vi "final.vi"() -> ()   [LabVIEW 2014]
panel:
  in  "start":bool
  out "Boolean":bool
  out "Score":i32
  out "XY Graph":cluster{dbl[], dbl[]}[](graph)
  in  "Width":dbl=6.0
  in  "stop":bool
  in  "UP":bool
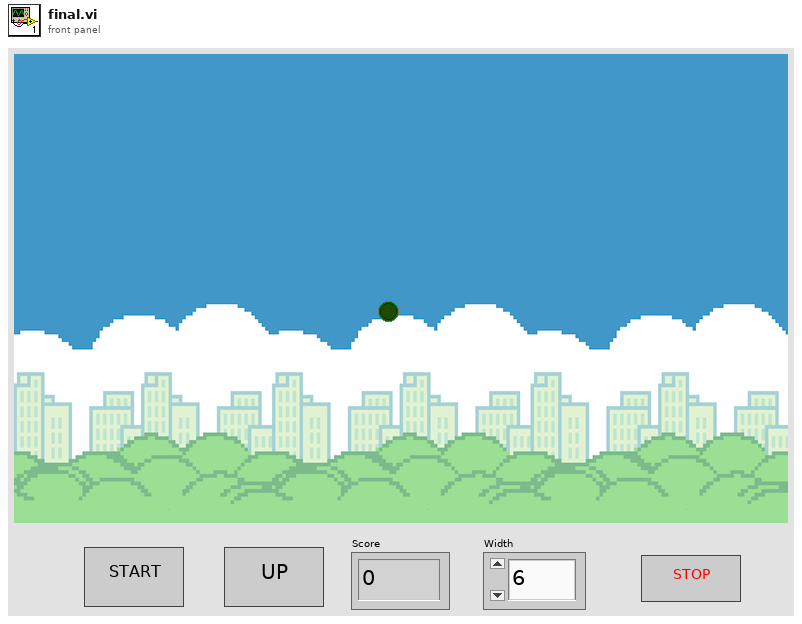
[diagram p1: front panel]
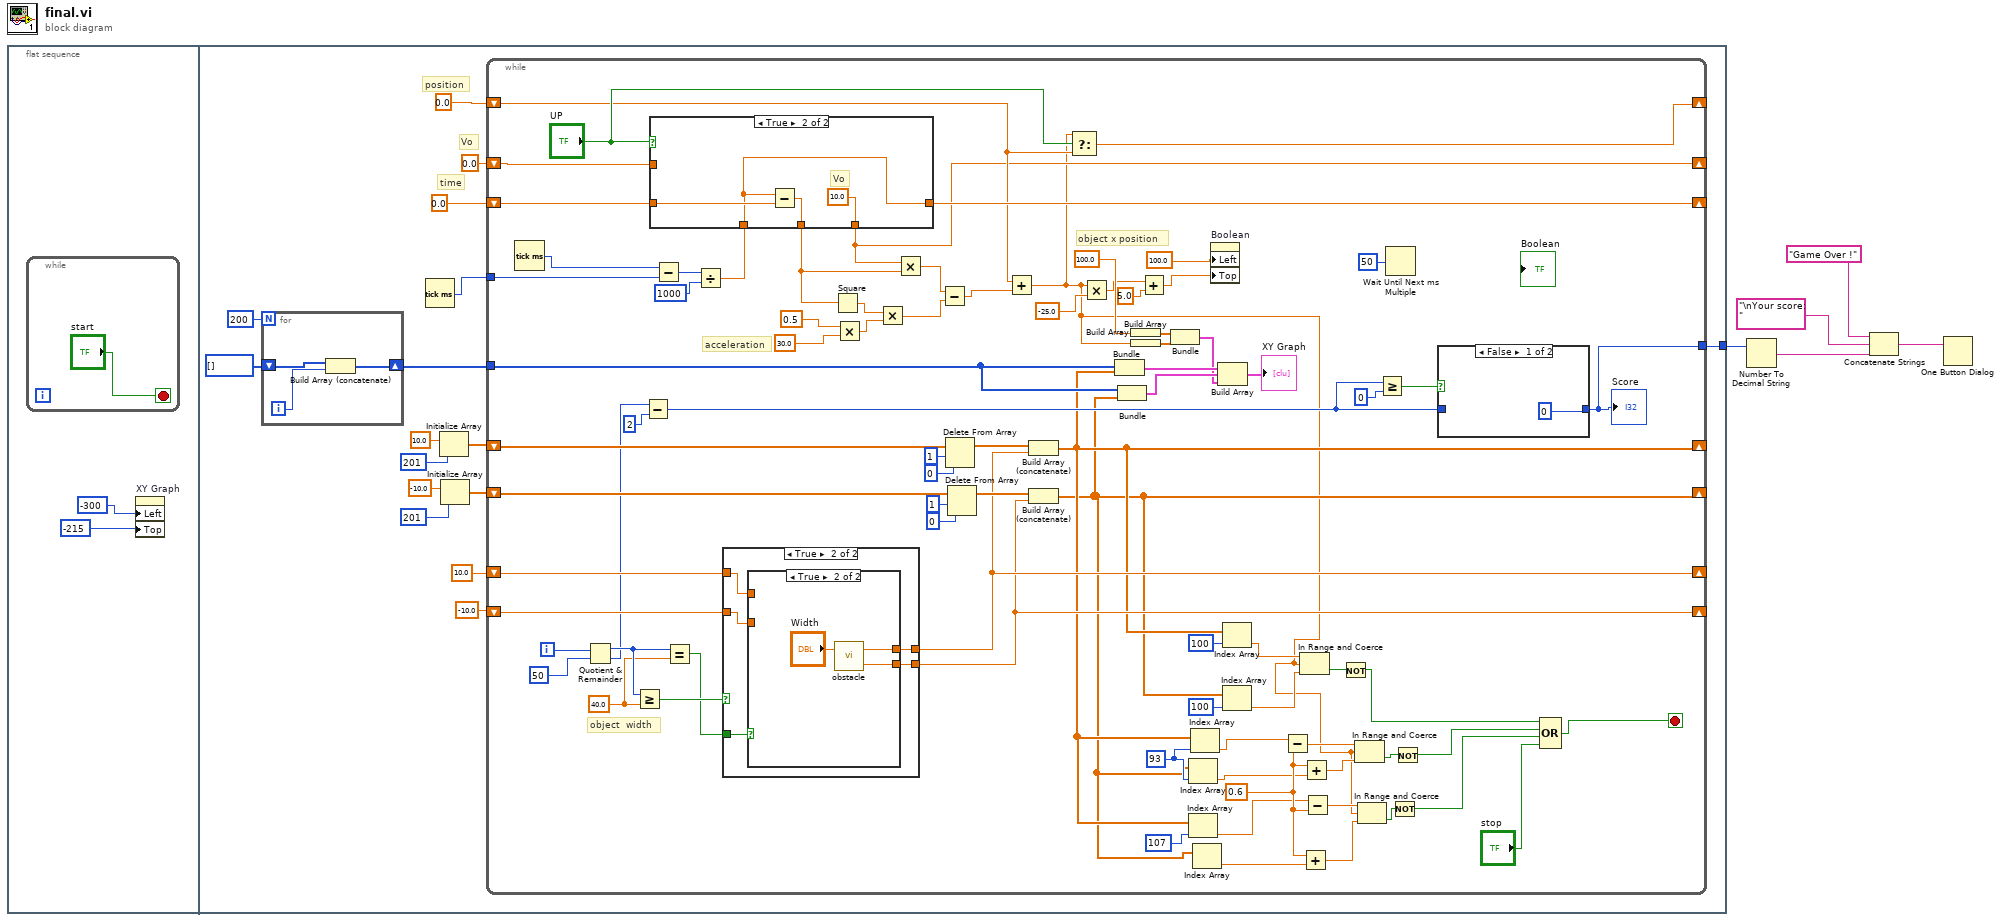
[diagram p0: block diagram]
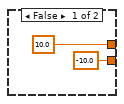
[diagram p3: hidden frame]
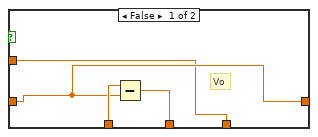
[diagram p5: hidden frame]
diagram:
  n1 = flat-sequence {
    tunnel: [w9] -> w4
    frame #0 {
      n2 = while {
        stop <- "start" stop-if-true
      }
      n3 = property on="XY Graph" class="XYGraph (strict)"("Left"=-300 ("Position:Left"), "Top"=-215 ("Position:Top")) -> ()  [unwired: 2 in, 2 out]
    }
    frame #1 {
      # "Vo"
      # "position"
      # "time"
      n4 = for {
        N: 200 -> [_]
        shift-right: [w25] -> w11
        shift-left: i32[] [] -> [w27]
        i -> [w26]
        n5 = Build Array (concatenate)(w27, w26) -> (w25:i32[])
      }
      n6 = Tick Count (ms)() -> (millisecond timer value=w22:u32)
      n7 = Initialize Array(10.0 ("element"), 201 ("dimension size")) -> (w17:dbl[])
      n8 = Initialize Array(-10.0 ("element"), 201 ("dimension size")) -> (w16:dbl[])
      n9 = while {
        shift-right: [w101] -> _
        shift-left: 0.0 -> [w106]
        tunnel: w22 -> [w110]
        shift-right: [w94] -> _
        shift-left: 0.0 -> [w95]
        shift-right: [w38] -> _
        shift-left: w17 -> [w90]
        shift-right: [w37] -> _
        shift-left: w16 -> [w89]
        shift-right: [w71] -> _
        shift-left: 10.0 -> [w81]
        shift-right: [w70] -> _
        shift-left: -10.0 -> [w80]
        tunnel: w11 -> [w77]
        shift-right: [w51] -> _
        shift-left: 0.0 -> [w52]
        tunnel: [w47] -> w9
        i -> [w92]
        stop <- w62 stop-if-true
        w39 = 0.6 ("y")
        w46 = 93 ("index")
        w61 = 40.0 ("y")
        # "object  width"
        # "object x position"
        # "acceleration"
        n10 = Tick Count (ms)() -> (millisecond timer value=w111:u32)
        n11 = Quotient & Remainder(x=w92, y=50) -> (x-y*floor(x/y)=w83:i32, floor(x/y)=w60:i32)
        n12 = Greater Or Equal?(x=w83, y=w61) -> (x >= y?=w84:bool)
        n13 = Subtract(x=w60, y=2) -> (x-y=w57:i32)
        n14 = Subtract(x=w111, y=w110) -> (x-y=w109:u32)
        n15 = Equal?(x=w83, y=w61) -> (x = y?=w82:bool)
        n16 = Divide(x=w109, y=u32 1000) -> (x/y=w107:dbl)
        n17 = case shown="True" "UP" {
          tunnel: w107 -> [w128 w131]
          tunnel: w106 -> [w127 w133]
          tunnel: [w129 w132] -> w100
          tunnel: [w127 w131] -> w101
          tunnel: [w126 10.0] -> w51
          tunnel: w52 -> [w126 _]
          frame False {
            # "Vo"
            n18 = Subtract(x=w128, y=w127) -> (x-y=w129:dbl)
          }
          frame True {
            # "Vo"
            n19 = Subtract(x=w131, y=w133) -> (x-y=w132:dbl)
          }
        }
        n20 = case shown="True" w84 {
          tunnel: w82 -> [_ w120]
          tunnel: w81 -> [_ w119]
          tunnel: w80 -> [_ w118]
          tunnel: [10.0 ("up") w117] -> w71
          tunnel: [-10.0 ("down") w116] -> w70
          frame False {
          }
          frame True {
            n21 = case shown="True" w120 {
              tunnel: w119 -> [w122 _]
              tunnel: w118 -> [w121 _]
              tunnel: [w122 w124] -> w117
              tunnel: [w121 w123] -> w116
              frame False {
              }
              frame True {
                n22 = call "obstacle.vi"("width"="Width") -> ("down"=w123:dbl, "up"=w124:dbl)  [unwired: 1 in]
              }
            }
          }
        }
        n23 = Square(x=w100) -> (x^2=w103:dbl)
        n24 = Multiply(x=0.5, y=30.0) -> (x*y=w102:dbl)
        n25 = Multiply(x=w103, y=w102) -> (x*y=w98:dbl)
        n26 = Multiply(x=w51, y=w100) -> (x*y=w99:dbl)
        n27 = Subtract(x=w99, y=w98) -> (x-y=w97:dbl)
        n28 = Delete From Array(array=w90, length=1, index=0) -> (array with subset deleted=w79:dbl[])  [unwired: 1 out]
        n29 = Delete From Array(array=w89, length=1, index=0) -> (array with subset deleted=w78:dbl[])  [unwired: 1 out]
        n30 = Add(x=w95, y=w97) -> (x+y=w31:dbl)
        n31 = Build Array (concatenate)(w79, w71) -> (w38:dbl[])
        n32 = Build Array (concatenate)(w78, w70) -> (w37:dbl[])
        n33 = Select(t=w31, s="UP", f=w95) -> (s? t:f=w94:dbl)
        n34 = Multiply(x=w31, y=-25.0) -> (x*y=w48:dbl)
        n35 = Bundle(w77, w38) -> (w76:cluster{i32[], dbl[]})  [unwired: 1 in]
        n36 = Bundle(w77, w37) -> (w75:cluster{i32[], dbl[]})  [unwired: 1 in]
        n37 = Build Array(100.0) -> (w74:dbl[])
        n38 = Build Array(w31) -> (w73:dbl[])
        n39 = Add(x=w48, y=5.0) -> (x+y=w49:dbl)
        n40 = Bundle(w74, w73) -> (w55:cluster{dbl[], dbl[]})  [unwired: 1 in]
        n41 = Index Array(array=w37, index=w46) -> (element=w35:dbl)
        n42 = Index Array(array=w38, index=107) -> (element=w34:dbl)
        n43 = Index Array(array=w38, index=w46) -> (element=w36:dbl)
        n44 = Index Array(array=w37) -> (element=w33:dbl)  [unwired: 1 in]
        n45 = property on="Boolean" class="Bool (strict)"("Left"=100.0, "Top"=w49) -> ()  [unwired: 2 in, 2 out]
        n46 = Build Array(w76, w75, w55) -> (→"XY Graph":cluster{dbl[], dbl[]}[])
        n47 = Index Array(array=w38, index=100) -> (element=w66:dbl)
        n48 = Index Array(array=w37, index=100) -> (element=w65:dbl)
        n49 = Subtract(x=w36, y=w39) -> (x-y=w42:dbl)
        n50 = In Range and Coerce(upper limit=w66, x=w31, lower limit=w65) -> (In Range?=w64:bool)  [unwired: 1 out]
        n51 = Add(x=w39, y=w33) -> (x+y=w32:dbl)
        n52 = Add(x=w39, y=w35) -> (x+y=w41:dbl)
        n53 = Subtract(x=w34, y=w39) -> (x-y=w40:dbl)
        n54 = Not(x=w64) -> (.not. x?=w63:bool)
        n55 = In Range and Coerce(upper limit=w42, x=w31, lower limit=w41) -> (In Range?=w43:bool)  [unwired: 1 out]
        n56 = In Range and Coerce(upper limit=w40, x=w31, lower limit=w32) -> (In Range?=w44:bool)  [unwired: 1 out]
        n57 = Greater Or Equal?(x=w57, y=0) -> (x >= y?=w58:bool)
        n58 = Wait Until Next ms Multiple(millisecond multiple=u32 50) -> ()  [unwired: 1 out]
        n59 = Not(x=w44) -> (.not. x?=w29:bool)
        n60 = Not(x=w43) -> (.not. x?=w30:bool)
        n61 = case shown="False" w58 {
          tunnel: w57 -> [_ w113]
          tunnel: [0 w113] -> w47
          frame False {
          }
          frame True {
          }
        }
        "Score" <- w47
        n62 = Compound Arithmetic op=OR(w63, w30, w29, "stop") -> (w62:bool)
      }
    }
  }
  n63 = Number To Decimal String(number=w4) -> (decimal integer string=w2:string)  [unwired: 1 in]
  n64 = Concatenate Strings("Game Over !" ("string"), "\nYour score: " ("string"), w2) -> (w5:string)
  n65 = One Button Dialog(message=w5) -> ()  [unwired: 1 in, 1 out]
